vi "Init.vi"(8 "error in":errorcluster, 11 "PCAN in":refnum<class "PCAN.lvclass">) -> (0 "error out":errorcluster, 3 "PCAN out":refnum<class "PCAN.lvclass">)   [LabVIEW 2024, in "PCAN.lvlib" / "PCAN.lvclass"]
uses:
  PCAN.lvclass
  PCAN.lvclass/PCAN.ctl
  <instrlib>/KDI Digital Instrumentation/API_for_PCAN_BASIC_FD/TPCANHandle.ctl
  <instrlib>/KDI Digital Instrumentation/API_for_PCAN_BASIC_FD/TPCANParameter.ctl
  <instrlib>/KDI Digital Instrumentation/API_for_PCAN_BASIC_FD/TPCANBaudrate.ctl
  <instrlib>/KDI Digital Instrumentation/API_for_PCAN_BASIC_FD/Error language selector.ctl
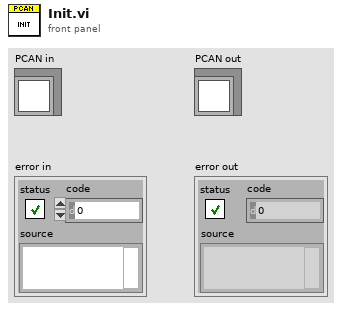
[diagram p1: front panel]
types:
  T1 = typedef "TPCANBaudrate.ctl" = enum16{"PCAN_BAUD_1M 0x0014", "PCAN_BAUD_800K 0x0016", "PCAN_BAUD_500K 0x001C", "PCAN_BAUD_250K 0x011C", "PCAN_BAUD_125K 0x031C", "PCAN_BAUD_100K 0x432F", "PCAN_BAUD_95K 0xC34E", "PCAN_BAUD_83K 0x852B", "PCAN_BAUD_50K 0x472F", "PCAN_BAUD_47K 0x1414", "PCAN_BAUD_33K 0x8B2F", "PCAN_BAUD_20K 0x532F", "PCAN_BAUD_10K 0x672F", "PCAN_BAUD_5K 0x7F7F", "User Baudrate"}
  T2 = typedef "TPCANHandle.ctl" = enum16{"PCAN_NONEBUS  0x000", "PCAN_ISABUS1  0x21", "PCAN_ISABUS2  0x22", "PCAN_ISABUS3  0x23", "PCAN_ISABUS4  0x24", "PCAN_ISABUS5  0x25", "PCAN_ISABUS6  0x26", "PCAN_ISABUS7  0x27", "PCAN_ISABUS8  0x28", "PCAN_DNGBUS1  0x31", "PCAN_PCIBUS1  0x41", "PCAN_PCIBUS1  0x42", "PCAN_PCIBUS1  0x43", "PCAN_PCIBUS1  0x44", "PCAN_PCIBUS1  0x45", "PCAN_PCIBUS1  0x46", "PCAN_PCIBUS1  0x47", "PCAN_PCIBUS1  0x48", "PCAN_PCIBUS1  0x409", "PCAN_PCIBUS1  0x40A", "PCAN_PCIBUS1  0x40B", "PCAN_PCIBUS1  0x40C", "PCAN_PCIBUS1  0x40D", "PCAN_PCIBUS1  0x40E", "PCAN_PCIBUS1  0x40F", "PCAN_PCIBUS1  0x410", "PCAN_USBBUS1  0x51", "PCAN_USBBUS2  0x52", "PCAN_USBBUS3  0x53", "PCAN_USBBUS4  0x54", "PCAN_USBBUS5  0x55", "PCAN_USBBUS6  0x56", "PCAN_USBBUS7  0x57", "PCAN_USBBUS8  0x58", "PCAN_USBBUS9  0x509", "PCAN_USBBUS10  0x50A", "PCAN_USBBUS11  0x50B", "PCAN_USBBUS12  0x50C", "PCAN_USBBUS13  0x50D", "PCAN_USBBUS14  0x50E", "PCAN_USBBUS15  0x50F", "PCAN_USBBUS16  0x510", "PCAN_PCCBUS1  0x61", "PCAN_PCCBUS2  0x62", "PCAN_LANBUS1  0x801", "PCAN_LANBUS2  0x802", "PCAN_LANBUS3  0x803", "PCAN_LANBUS4  0x804", "PCAN_LANBUS5  0x805", "PCAN_LANBUS6  0x806", "PCAN_LANBUS7  0x807", "PCAN_LANBUS8  0x808", "PCAN_LANBUS9  0x809", "PCAN_LANBUS10  0x80A", "PCAN_LANBUS11  0x80B", "PCAN_LANBUS12  0x80C", "PCAN_LANBUS13  0x80D", "PCAN_LANBUS14  0x80E", "PCAN_LANBUS15  0x80F", "PCAN_LANBUS16  0x810"}
  T3 = typedef "TPCANParameter.ctl" = enum8{"Not Available", "PCAN device number", "PCAN 5-volt power", "PCAN receive event", "PCAN message filter", "PCAN API version", "PCAN channel version", "PCAN busoff autoreset", "PCAN listen-only", "PCAN log location", "PCAN log status", "PCAN log configure", "PCAN log text", "PCAN channel condition", "PCAN hardware name", "PCAN_RECEIVE_STATUS", "PCAN_CONTROLLER_NUMBER", "PCAN_TRACE_LOCATION ", "PCAN_TRACE_STATUS", "PCAN_TRACE_SIZE", "PCAN_TRACE_CONFIGURE", "PCAN_CHANNEL_IDENTIFYING", "PCAN_CHANNEL_FEATURES", "PCAN_SPEED_ADAPTING", "PCAN_BITRATE_INFO", "PCAN_BITRATE_INFO_FD", "PCAN_BUSSPEED_NOMINAL", "PCAN_BUSSPEED_DATA", "PCAN_IP_ADDRESS", "PCAN_LAN_SERVICE_STATUS", "PCAN_ALLOW_STATUS_FRAMES", "PCAN_ALLOW_RTR_FRAMES", "PCAN_ALLOW_ERROR_FRAMES", "PCAN_INTERFRAME_DELAY", "PCAN_ACCEPTANCE_FILTER_11BIT", "PCAN_ACCEPTANCE_FILTER_29BIT", "PCAN_IO_DIGITAL_CONFIGURATION", "PCAN_IO_DIGITAL_VALUE", "PCAN_IO_DIGITAL_SET", "PCAN_IO_DIGITAL_CLEAR", "PCAN_IO_ANALOG_VALUE", "PCAN_FIMRWARE_VRSION", "PCAN__ATTACHED_CHANNELS_COUNT", "PCAN_ATTACHED CHANNELS"}
  T4 = typedef "Error language selector.ctl" = u16
  T5 = typedef "Channel Availability.ctl" = enum16{"PCAN_CHANNEL_UNAVAILABLE", "PCAN_CHANNEL_AVAILABLE", "PCAN_CHANNEL_OCCUPIED", "PCAN_CHANNEL_PCANVIEW "}
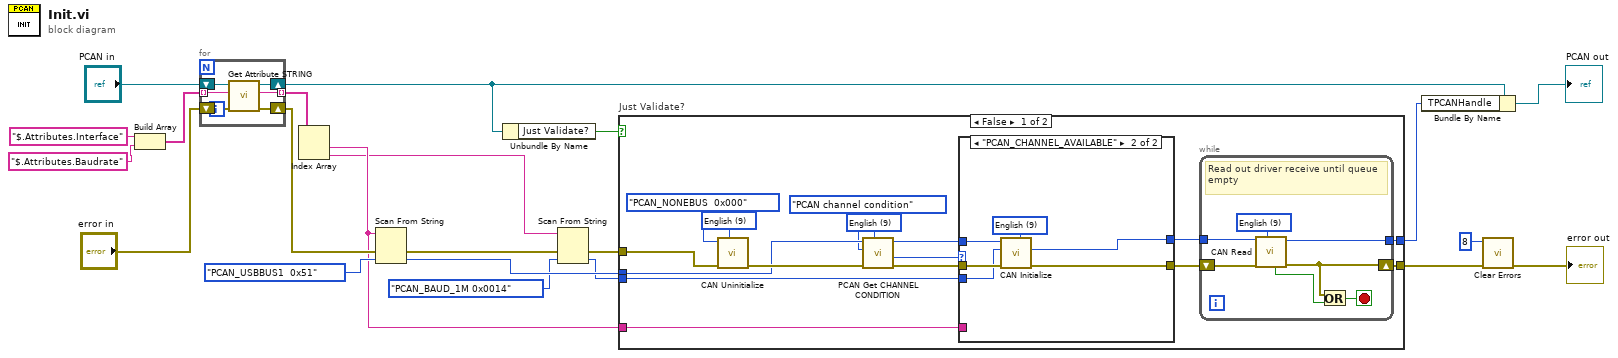
[diagram p0: block diagram]
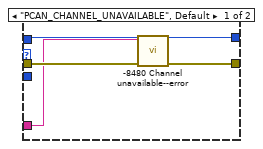
[diagram p2: hidden frame]
diagram:
  n1 = Build Array("$.Attributes.Interface" ("Attribute"), "$.Attributes.Baudrate" ("Attribute")) -> (w1:string[])
  n2 = for {
    tunnel: [w28] -> w18 mode=indexing
    tunnel: w1 -> [w23] mode=indexing
    shift-right: [w24] -> w5
    shift-left: "PCAN in" -> [w27]
    shift-right: [w25] -> w9
    shift-left: "error in" -> [w26]
    n3 = call-dynamic "Get Attribute STRING.vi"("error in"=w26, "Attribute"=w23, "IConfigurable in"=w27) -> ("error out"=w25:errorcluster, "Value"=w28:string, "IConfigurable out"=w24:refnum<class "PCAN.lvclass">)  [unwired: 6 in]
  }
  n4 = Index Array(array=w18) -> (element #1=w8:string, element #2=w7:string)  [unwired: 2 in]
  n5 = Scan From String(input string=w8, error in=w9, default 1=TPCANHandle."PCAN_USBBUS1  0x51" ("TPCANHandle")) -> (error out=w6:errorcluster, output 1=w20:T2)  [unwired: 2 in, 2 out]
  n6 = Unbundle By Name(w5) -> ("Just Validate?"=w4:bool)
  n7 = Scan From String(input string=w7, error in=w6, default 1=TPCANBaudrate."PCAN_BAUD_1M 0x0014" ("TPCANBaudrate")) -> (error out=w17:errorcluster, output 1=w16:T1)  [unwired: 2 in, 2 out]
  n8 = case "Just Validate?" shown="False" w4 {
    tunnel: w20 -> [w42 _]
    tunnel: w8 -> [w41 _]
    tunnel: w17 -> [w40 w62]
    tunnel: w16 -> [w39 _]
    tunnel: [w37 w62] -> w14
    tunnel: [w36 _] -> w13
    frame False {
      w29 = T4 9 items=["System dependent", "Not available", "Not available", "Not available", "Not available", "Not available", "Not available", "Deutsch", "Not available", "English", "Español", "Not available", "Français", "Not available", "Not available", "Not available", "Italiano"] ("Language")
      w38 = T4 9 items=["System dependent", "Not available", "Not available", "Not available", "Not available", "Not available", "Not available", "Deutsch", "Not available", "English", "Español", "Not available", "Français", "Not available", "Not available", "Not available", "Italiano"] ("Language")
      n9 = call <instrlib>:"CAN Uninitialize.vi"("Language"=w38, "error in (no error)"=w40, "TPCANHandle"=TPCANHandle."PCAN_NONEBUS  0x000") -> ("error out"=w44:errorcluster)  [unwired: 6 in, 2 out]
      n10 = call <instrlib>:"PCAN Get CHANNEL CONDITION.vi"("Language"=w29, "error in (no error)"=w44, "TPCANParameter"=TPCANParameter."PCAN channel condition", "TPCANHandle"=w42) -> ("error out"=w35:errorcluster, "Channel condition"=w34:T5, "TPCANHandle out"=w33:T2)  [unwired: 5 in]
      n11 = case shown="\"PCAN_CHANNEL_AVAILABLE\"" w34 {
        tunnel: w35 -> [w47 w54]
        tunnel: [w48 w53] -> w32
        tunnel: w33 -> [w46 w52]
        tunnel: [w46 w51] -> w31
        tunnel: w41 -> [w45 _]
        tunnel: w39 -> [_ w50]
        frame "PCAN_CHANNEL_UNAVAILABLE", Default {
          n12 = call "-8480 Channel unavailable--error.vi"("error in (no error)"=w47, "Channel"=w45) -> ("error out"=w48:errorcluster)  [unwired: 9 in]
        }
        frame "PCAN_CHANNEL_AVAILABLE" {
          w49 = T4 9 items=["System dependent", "Not available", "Not available", "Not available", "Not available", "Not available", "Not available", "Deutsch", "Not available", "English", "Español", "Not available", "Français", "Not available", "Not available", "Not available", "Italiano"] ("Language")
          n13 = call <instrlib>:"CAN Initialize.vi"("Language"=w49, "error in (no error)"=w54, "TPCANBaudrate"=w50, "TPCANHandle"=w52) -> ("error out"=w53:errorcluster, "TPCANHandle_out"=w51:T2)  [unwired: 5 in, 1 out]
        }
      }
      n14 = while {
        shift-right: [w59] -> w37
        shift-left: w32 -> [w61]
        tunnel: w31 -> [w57]
        tunnel: [w56] -> w36
        stop <- w60 stop-if-true
        w55 = T4 9 items=["System dependent", "Not available", "Not available", "Not available", "Not available", "Not available", "Not available", "Deutsch", "Not available", "English", "Español", "Not available", "Français", "Not available", "Not available", "Not available", "Italiano"] ("Language")
        # "Read out driver receive until queue empty"
        n15 = call <instrlib>:"CAN Read.vi"("Language"=w55, "error in (no error)"=w61, "TPCANHandle"=w57) -> ("error out"=w59:errorcluster, "TPCANHandle out"=w56:T2, "rcv queue empty"=w58:bool)  [unwired: 4 in, 2 out]
        n16 = Or(x=w59, y=w58) -> (x .or. y?=w60:bool)
      }
    }
    frame True {
    }
  }
  n17 = Bundle By Name(cluster=w5, "TPCANHandle"=w13) -> (→"PCAN out":refnum<class "PCAN.lvclass">)
  n18 = call <vilib>:"Clear Errors.vi"("error in (no error)"=w14, "specific error code to clear (0: all)"=8) -> ("error out"=→"error out":errorcluster)  [unwired: 4 in, 1 out]
